vi "Int32 Create.vi"(8 "error in (no error)":errorcluster, 11 "I32 in":i32) -> (0 "error out":errorcluster, 3 "Int32 DVR out":refnum<data-value>)   [LabVIEW 2015, in "MDSplus.lvlib"]
uses:
  MDSplus.lvlib
  Classes/Data_Class/Scalar_Class/Int32_Class/Int32.lvclass
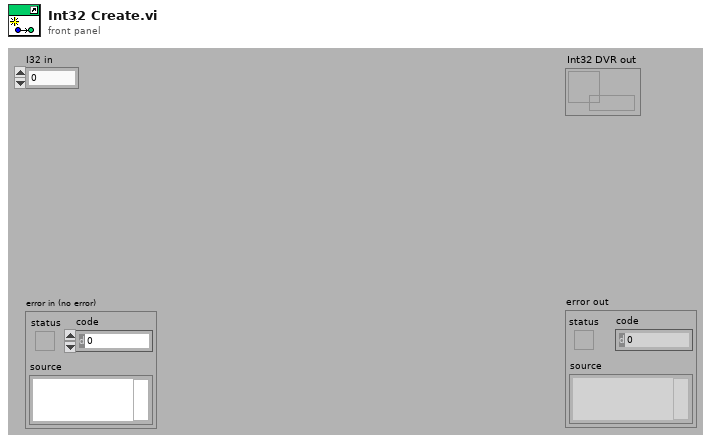
[diagram p1: front panel]
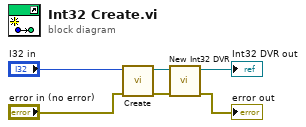
[diagram p0: block diagram]
diagram:
  n1 = call "Create.vi"("error in (no error)"="error in (no error)", "I32 in"="I32 in") -> ("error out"=w3:errorcluster, "Int32 out"=w4:refnum<class "Int32.lvclass">)  [unwired: 8 in]
  n2 = call "New Int32 DVR.vi"("error in (no error)"=w3, "Int32 in"=w4) -> ("error out"=→"error out":errorcluster, "Int32 DVR out"=→"Int32 DVR out":refnum<data-value>)  [unwired: 8 in]
